vi "编码规则设置.vi"() -> ()   [LabVIEW 2020]
panel:
  in  "更多正则表达式":bool
  in  "正则表达式简单说明":bool
  in  "?":string
  # "编码规则"
  # "注意事项：\n1、编码规则采用正则表达式。\n2、编码规则区分大小写。\n3、每行对应一条编码规则，每行编码规则之间为“或”关系。\n4、编码规则之间不要留有空行。"
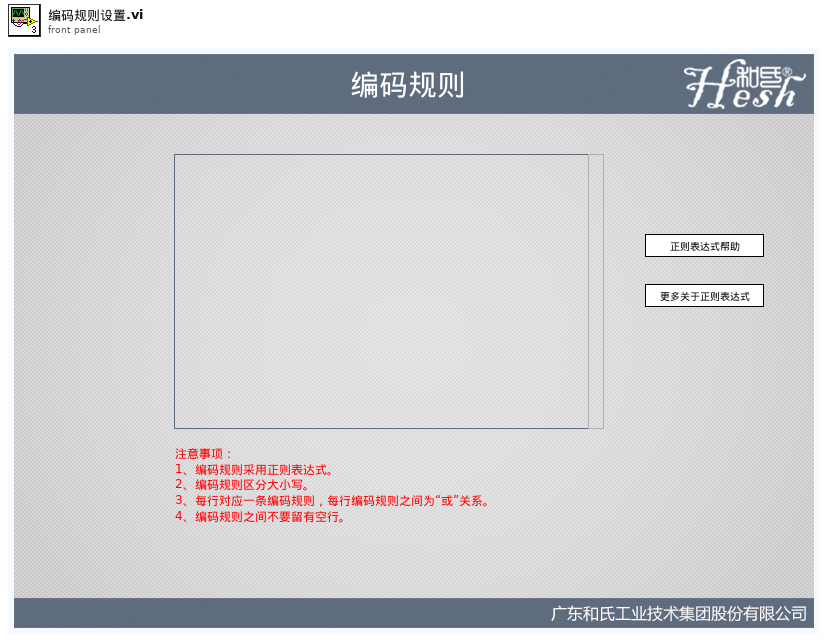
[diagram p1: front panel]
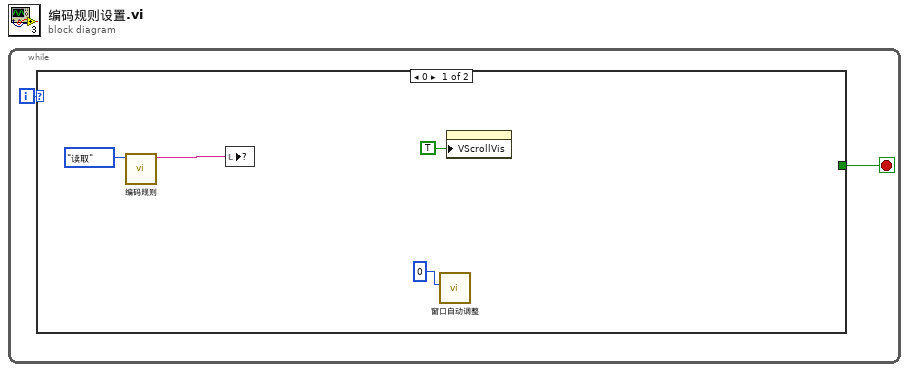
[diagram p0: block diagram]
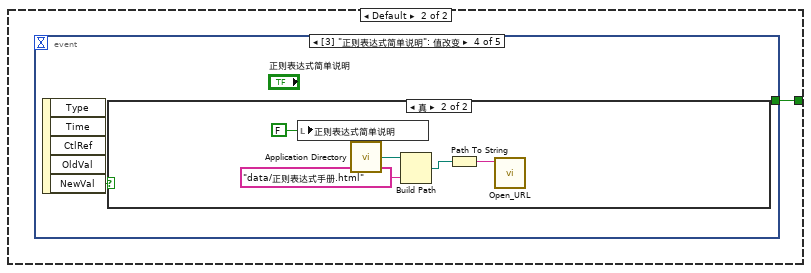
[diagram p2: hidden frame]
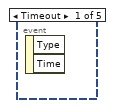
[diagram p3: hidden frame]
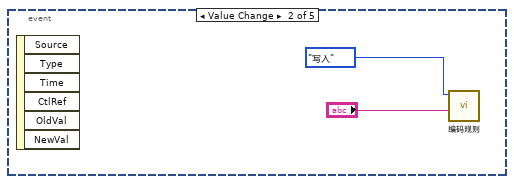
[diagram p4: hidden frame]
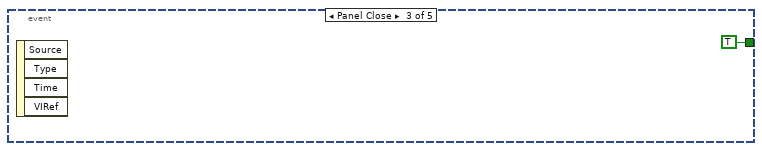
[diagram p5: hidden frame]
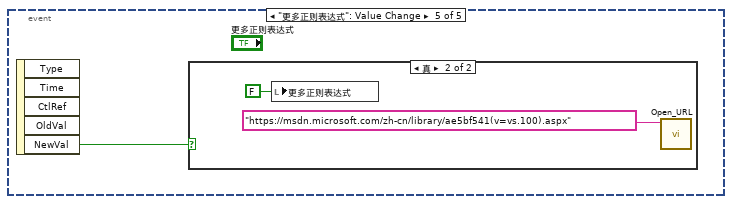
[diagram p7: hidden frame]
diagram:
  n1 = while {
    i -> [w1]
    stop <- w2 stop-if-true
    n2 = case shown="0" w1 {
      tunnel: [_ w7] -> w2
      frame 0 {
        n3 = call "编码规则.vi"("功能"=enum16{"读取", "写入"}."读取") -> ("正则表达式输出（单行）"=w5:string)  [unwired: 8 in, 2 out]
        n4 = local write item#?(w5) -> ()
        n5 = call "窗口自动调整.vi"("border spacing (2 px)"=0) -> ()  [unwired: 5 in, 2 out]
        n6 = property class="Str"("VScrollVis"=TRUE ("垂直滚动条可见")) -> ()  [unwired: 2 in, 2 out]
      }
      frame Default {
        n7 = event shown="[3] \"正则表达式简单说明\": 值改变" {
          selector: _ -> [_ _ _ _ _]
          dyn-events: _ -> [_ _ _ _ _]
          timeout: _ -> [_ _ _ _ _]
          tunnel: [_ _ TRUE _ _] -> w7
          event Timeout {
            n8 = event-data() -> ()  [unwired: 1 in, 2 out]
          }
          event Value Change {
            n9 = event-data() -> ()  [unwired: 1 in, 6 out]
            n10 = call "编码规则.vi"("编码正则表达式"="?", "功能"=enum16{"读取", "写入"}."写入") -> ()  [unwired: 7 in, 3 out]
          }
          event Panel Close {
            n11 = event-data() -> ()  [unwired: 1 in, 4 out]
          }
          event "正则表达式简单说明": Value Change {
            n12 = event-data() -> ("NewVal"=w11:bool)  [unwired: 1 in, 4 out]
            n13 = case shown="真" w11 {
              frame False {
              }
              frame True {
                n14 = local write "正则表达式简单说明"(FALSE ("正则表达式简单说明")) -> ()
                n15 = call <vilib>:"Application Directory.vi"() -> ("Application Directory"=w14:path)
                n16 = Build Path(base path=w14, name or relative path="data/正则表达式手册.html" ("名称或相对路径")) -> (appended path=w12:path)
                n17 = Path To String(path=w12) -> (string=w15:string)
                n18 = call "Open_URL.vi"("URL"=w15) -> ()  [unwired: 11 in]
              }
            }
          }
          event "更多正则表达式": Value Change {
            n19 = event-data() -> ("NewVal"=w17:bool)  [unwired: 1 in, 4 out]
            n20 = case shown="真" w17 {
              frame False {
              }
              frame True {
                n21 = local write "更多正则表达式"(FALSE ("更多正则表达式")) -> ()
                n22 = call "Open_URL.vi"("URL"="https://msdn.microsoft.com/zh-cn/library/ae5bf541(v=vs.100).aspx" ("command line")) -> ()  [unwired: 11 in]
              }
            }
          }
        }
      }
    }
  }
